vi "Pockels Cal-Header strings.vi"() -> (1 "Cal data header string":string="Cal data", 2 "Cal subset indexes header string":string, 3 "Cal wavelength string":string)   [LabVIEW 2017]
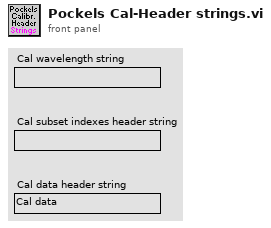
[diagram p1: front panel]
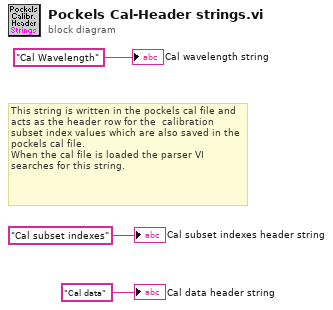
[diagram p0: block diagram]
diagram:
  # "This string is written in the pockels cal file and acts as the header row for the  calibration subset index values which are also saved in the pockels cal file.\nWhen the cal file is loaded the parser VI searches for this string."
  "Cal subset indexes header string" <- "Cal subset indexes" ("element")
  "Cal wavelength string" <- "Cal Wavelength" ("element")
  "Cal data header string" <- "Cal data" ("Cal data header row")
